vi "ProcessData.vi"(8 "error in (no error)":errorcluster, 9 "State":T1, 10 "Analog Data":T3, 11 "MultDimExperiment in":refnum<class "MultDimExperiment.lvclass">) -> (0 "error out":errorcluster, 1 "Fixated":bool, 2 "Trigger":T2=enum."Broke Fixation", 3 "MultDimExperiment out":refnum<class "MultDimExperiment.lvclass">)   [LabVIEW 2010]
uses:
  Core SubVIs/Core SubVIs.lvlib
  <vilib>/measure/NI_MAPro.lvlib
  <vilib>/measure/madcrms.llb/Basic Averaged DC-RMS for 1 Chan.vi
  Trial Based Experiment Statechart/Trial Based Experiment.lvsc/Trigger.ctl
  Trial Based Experiment Statechart/Trial Based Experiment.lvsc
  Trial Based Experiment Statechart/Trial Based Experiment.lvsc/State.ctl
  MultDimExperiment.lvclass
  Core SubVIs/Controls/TYPE - Analog Data.ctl
panel:
  in  "Adjustment Rate":dbl=0.02
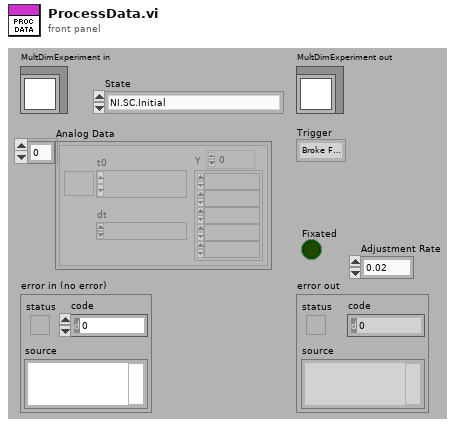
[diagram p1: front panel]
types:
  T1 = typedef "Trial Based Experiment.lvsc/State.ctl" = enum16{"NI.SC.Initial", "NI.SC.History", "NI.SC.ShallowHistory", "NI.SC.Terminal", "Cleanup", "State", "State\\Region\\Pause", "State\\Region\\Response Period", "State\\Region\\Delay Period", "State\\Region\\Hold Fixation", "State\\Region\\Acquire Fixation", "State\\Region\\Abort Trial", "State\\Region\\End Trial", "State\\Region\\Intertrial", "State\\Region\\Start Trial"}
  T2 = typedef "Trial Based Experiment.lvsc/Trigger.ctl" = enum16{"NULL", "Fixated", "Broke Fixation", "Stop", "Correct Response", "Incorrect Response", "Timeout"}
  T3 = typedef "Core SubVIs.lvlib/TYPE - Analog Data.ctl" = waveform(dbl)[]
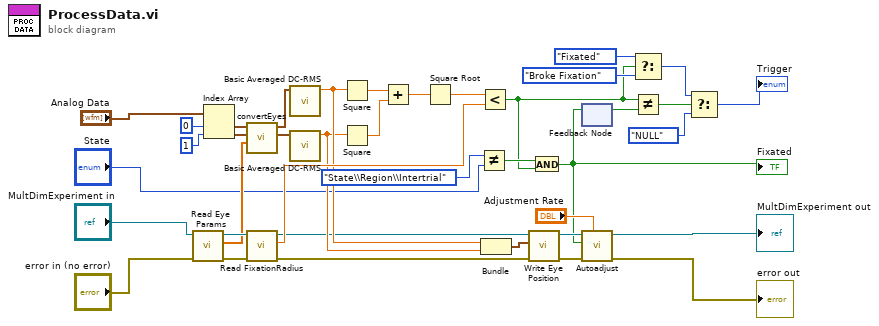
[diagram p0: block diagram]
diagram:
  n1 = call-dynamic "Read Eye Params.vi"("error in (no error)"="error in (no error)", "TrialBasedExperiment in"="MultDimExperiment in") -> ("error out"=w20:errorcluster, "Eye Params"=w33:dbl[], "TrialBasedExperiment out"=w39:refnum<class "MultDimExperiment.lvclass">)  [unwired: 7 in]
  n2 = Index Array(array="Analog Data", index #1=0 ("index"), index #2=1 ("index")) -> (element #1=w32:waveform(dbl), element #2=w31:waveform(dbl))
  n3 = call "convertEyes.vi"("Params"=w33, "Vertical"=w31, "Horizontal"=w32) -> ("Vertical Calibrated"=w36:waveform(dbl), "Horizontal Calibrated"=w35:waveform(dbl))  [unwired: 7 in]
  n4 = call-dynamic "Read FixationRadius.vi"("error in (no error)"=w20, "MatlabExperiment in"=w39) -> ("error out"=w13:errorcluster, "FixationRadius"=w21:dbl, "MatlabExperiment out"=w16:refnum<class "MultDimExperiment.lvclass">)  [unwired: 7 in]
  n5 = call-poly <vilib>:"Basic Averaged DC-RMS.vi"("signal in"=w35) -> ("DC value"=w19:dbl)  [unwired: 7 in, 3 out]
  n6 = call-poly <vilib>:"Basic Averaged DC-RMS.vi"("signal in"=w36) -> ("DC value"=w18:dbl)  [unwired: 7 in, 3 out]
  n7 = Square(x=w19) -> (x^2=w27:dbl)
  n8 = Square(x=w18) -> (x^2=w26:dbl)
  n9 = Add(x=w27, y=w26) -> (x+y=w25:dbl)
  n10 = Square Root(x=w25) -> (sqrt(x)=w24:dbl)
  n11 = Not Equal?(x=State."State\\Region\\Intertrial", y="State") -> (x != y?=w10:bool)
  n12 = Less?(x=w24, y=w21) -> (x < y?=w9:bool)
  n13 = Bundle("DC value"=w19, "DC value"=w18) -> (w17:cluster{"DC value":dbl, "DC value":dbl})  [unwired: 1 in]
  n14 = call-dynamic "Write Eye Position.vi"("error in (no error)"=w13, "Eye Position"=w17, "TrialBasedExperiment in"=w16) -> ("error out"=w12:errorcluster, "TrialBasedExperiment out"=w15:refnum<class "MultDimExperiment.lvclass">)  [unwired: 7 in]
  n15 = And(x=w10, y=w9) -> (x .and. y?=w4:bool)
  "Fixated" <- w4
  n16 = feedback #1() -> (w28:bool)  [unwired: 1 in]
  n17 = feedback-in #1(w4) -> ()
  n18 = call-dynamic "Autoadjust.vi"("Adjustment Rate"="Adjustment Rate", "error in (no error)"=w12, "Fixated"=w4, "TrialBasedExperiment in"=w15) -> ("error out"=→"error out":errorcluster, "TrialBasedExperiment out"=→"MultDimExperiment out":refnum<class "MultDimExperiment.lvclass">)  [unwired: 6 in]
  n19 = Select(t=Trigger."Fixated" ("Trigger"), s=w9, f=Trigger."Broke Fixation" ("Trigger")) -> (s? t:f=w29:T2)
  n20 = Not Equal?(x=w9, y=w28) -> (x != y?=w22:bool)
  n21 = Select(t=w29, s=w22, f=Trigger."NULL" ("Trigger")) -> (s? t:f=→"Trigger":T2)
